vi "Security.MasterKeyChannelValues.Get.vi"(8 "error in (no error)":errorcluster, 11 "Device Item Ref in":T1 format="%.0x") -> (0 "error out":errorcluster, 2 "MasterKey":string, 3 "Section Ref out":T1 format="%.0x")   [LabVIEW 2019, in "Diagnostics Addon System Explorer.lvlib"]
uses:
  Diagnostics Addon System Explorer.lvlib
  <vilib>/NI VeriStand/Custom Device API/Custom Device Item Ref.ctl
  Addon Shared/SubVIs/Constants.vi
  <vilib>/NI VeriStand/Custom Device Tools/Custom Device Utility Library/NI VeriStand - Search for Item by GUID.vi
  <vilib>/NI VeriStand/Custom Device Tools/Custom Device Utility Library/NI VeriStand - Search for Item by Name.vi
  <vilib>/NI VeriStand/Custom Device Tools/Custom Device Utility Library/Custom Device Utility Library.lvlib
  Addon Shared/Diagnostics Addon Shared.lvlib
  <vilib>/NI VeriStand/Custom Device API/Custom Device API.lvlib
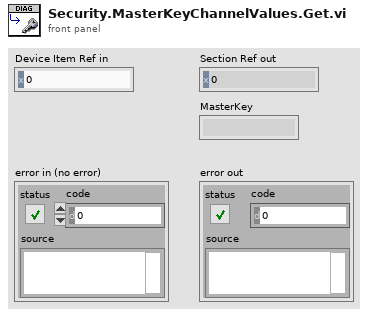
[diagram p1: front panel]
types:
  T1 = typedef "Custom Device API.lvlib/Custom Device Item Ref.ctl" = u64
  T2 = typedef "Custom Device API.lvlib/Custom Device Channel.ctl" = cluster{"Type":T3, "Units":string, "Default Value":dbl, "Faultable":bool, "Scalable":bool}
  T3 = typedef "Custom Device API.lvlib/Custom Device Channel Type.ctl" = enum16{"Input", "Output"}
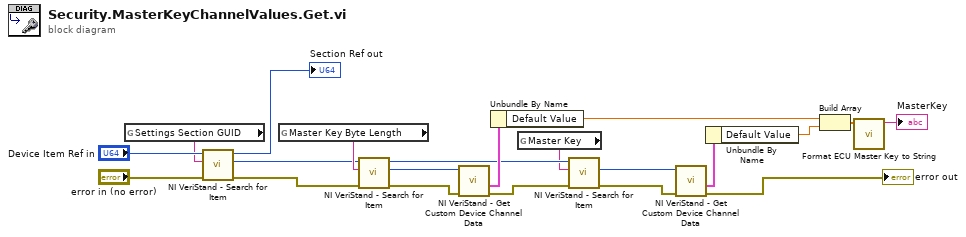
[diagram p0: block diagram]
diagram:
  n1 = global read "Constants.vi" "Settings Section GUID"() -> (w2:string)
  n2 = call-poly <vilib>:"NI VeriStand - Search for Item.vi"("error in"="error in (no error)", "Item GUID"=w2, "Section Ref in"="Device Item Ref in") -> ("error out"=w4:errorcluster, "Item Ref"=w3:T1, "Section Ref out"=→"Section Ref out":T1)  [unwired: 5 in, 1 out]
  n3 = global read "Constants.vi" "Master Key Byte Length"() -> (w5:string)
  n4 = call-poly <vilib>:"NI VeriStand - Search for Item.vi"("error in"=w4, "Item Name"=w5, "Section Ref in"=w3) -> ("error out"=w13:errorcluster, "Item Ref"=w12:T1, "Section Ref out"=w9:T1)  [unwired: 5 in, 1 out]
  n5 = call <vilib>:"NI VeriStand - Get Custom Device Channel Data.vi"("error in (no error)"=w13, "Channel Ref in"=w12) -> ("error out"=w14:errorcluster, "Channel"=w15:T2)  [unwired: 4 in, 4 out]
  n6 = Unbundle By Name(w15) -> ("Default Value"=w19:dbl)
  n7 = global read "Constants.vi" "Master Key"() -> (w8:string)
  n8 = call-poly <vilib>:"NI VeriStand - Search for Item.vi"("error in"=w14, "Item Name"=w8, "Section Ref in"=w9) -> ("error out"=w10:errorcluster, "Item Ref"=w11:T1)  [unwired: 5 in, 2 out]
  n9 = call <vilib>:"NI VeriStand - Get Custom Device Channel Data.vi"("error in (no error)"=w10, "Channel Ref in"=w11) -> ("error out"=→"error out":errorcluster, "Channel"=w16:T2)  [unwired: 4 in, 4 out]
  n10 = Unbundle By Name(w16) -> ("Default Value"=w18:dbl)
  n11 = Build Array(w19, w18) -> (w20:dbl[])
  n12 = call "Format ECU Master Key to String.vi"("Data"=w20) -> ("string"=→"MasterKey":string)  [unwired: 10 in]
